vi "X-CAN_Connection_Stream_Connection.vi"() -> ()   [LabVIEW 2015]
uses:
  <vilib>/Stratom, Inc/X-CAN for myRIO (API)/X-CAN Class/Type Definitions/CAN_Speed.ctl
  <vilib>/Stratom, Inc/X-Modules for myRIO/Type Defs/MXPChannel.ctl
  <vilib>/Platform/TimedLoop/XDataNode/timing_clust.ctl
  <vilib>/Platform/TimedLoop/XDataNode/nitl_modes.ctl
  <vilib>/Platform/TimedLoop/XDataNode/wakeup.ctl
  <vilib>/platform/TimedLoop/XDataNode/XDataNode.xnode
  <vilib>/Stratom, Inc/X-CAN for myRIO (API)/X-CAN Class/X-CAN.lvclass
  <vilib>/Platform/TimedLoop/XDataNode/XDNodeRunTimeDep.lvlib
panel:
  out "Motor positions (degree)":T1(array[cluster]) {"Error Code (bits)" format="%b"}
  in  "Stop Button":bool
  # "REMEMBER: this subVI has always to be run as first."
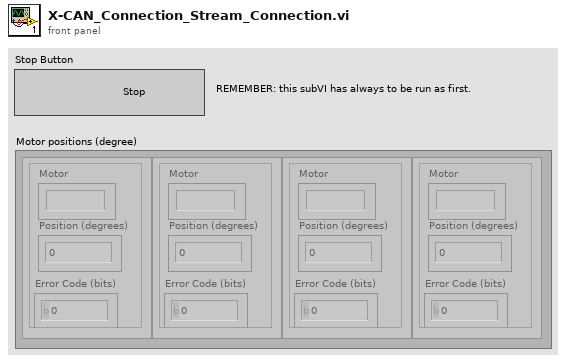
[diagram p1: front panel]
types:
  T1 = cluster{"Position (degrees)":i32, "Error Code (bits)":u8, "Motor":string}[]
  T2 = cluster{"Desired Position":u16, "Enable?":bool, "Reset?":bool}[]
  T3 = typedef "MXPChannel.ctl" = enum16{"A/MXP", "B/MXP"}
  T4 = typedef "X-CAN.lvclass/CAN_Speed.ctl" = u8
  T5 = cluster{"ID":u8, "Position":u16, "Error Code":u8}[]
  T6 = typedef "XDNodeRunTimeDep.lvlib/timing_clust.ctl" = cluster{"Expected End [f-1]":u64, "Actual End [f-1]":u64, "Finished Late? [f-1]":bool, "Expected End [i-1]":u64, "Actual End [i-1]":u64, "Finished Late? [i-1]":bool, "Expected Start [i]":u64, "Actual Start [i]":u64, "Expected Start [f]":u64, "Actual Start [f]":u64, "Source Name":string, "Structure Name":string, "Period":i64, "Deadline":i64, "Offset":i64, "Start":i64, "Priority":i32, "Timeout":i32, "Mode":T7, "Wakeup Reason":T8, "Error":errorcluster, "Source Type":string, "Secondary Source Type":string, "Global End Time":u64, "Global Start Time":u64, "Frame Duration":u64, "Iteration Duration":u64, "Assigned CPU":i32, "I/O Scan Engine Mode":u32}
  T7 = typedef "XDNodeRunTimeDep.lvlib/nitl_modes.ctl" = enum32{"No Change", "Process missed periods, maintain original phase", "Discard missed periods, maintain original phase", "Process missed periods, ignore original phase", "Discard missed periods, ignore original phase"}
  T8 = typedef "XDNodeRunTimeDep.lvlib/wakeup.ctl" = enum32{"Normal", "Aborted", "Asynchronous wakeup", "Timing source error", "Timed loop error", "Timeout"}
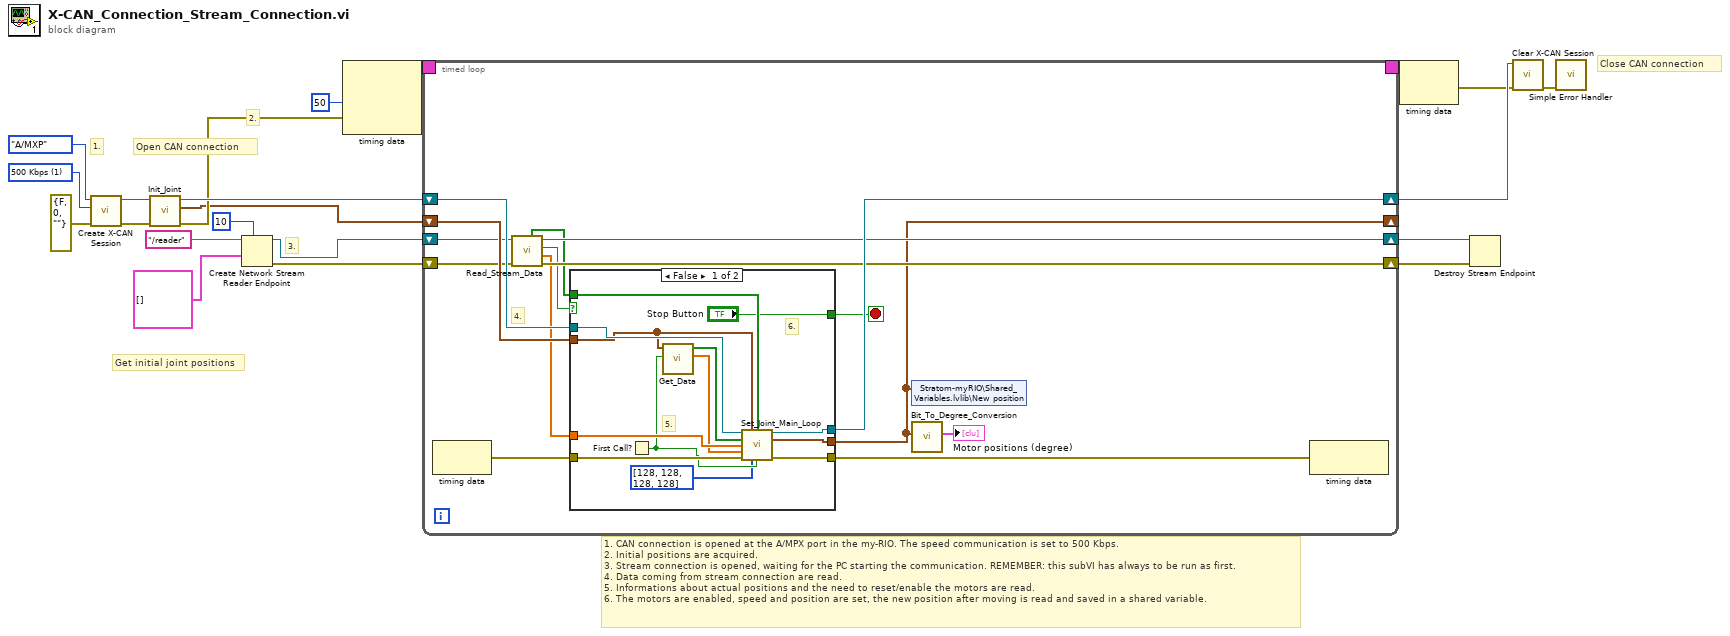
[diagram p0: block diagram]
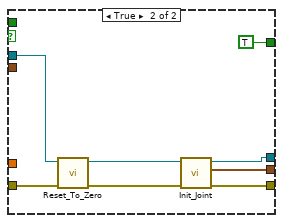
[diagram p2: hidden frame]
diagram:
  w20 = T4 1 items=["125 Kbps"=7, "250 Kbps"=3, "500 Kbps"=1, "1000 Kbps"=0, "95.238 Kbps"=6] ("CAN Speed [Kbps]")
  # "Close CAN connection"
  # "3."
  # "2."
  # "1."
  # "1. CAN connection is opened at the A/MPX port in the my-RIO. The speed communication is set to 500 Kbps.\n2. Initial positions are acquired.\n3. Stream connection is opened, waiting for the PC starting the communication. REMEMBER: this subVI has always to be run as first. \n4. Data coming from stream connection are read.\n5. Informations about actual positions and the need to reset/enable the motors are read.\n6. The motors are enabled, speed and position are set, the new position after moving is read and saved in a shared variable."
  # "Get initial joint positions"
  # "Open CAN connection"
  n1 = call <vilib>:"Create X-CAN Session.vi"("error in (no error)"=errorcluster {"status"=FALSE, "code"=0, "source"=""}, "CAN Speed [Kbps]"=w20, "MXP Channel"=MXPChannel."A/MXP") -> ("error out"=w11:errorcluster, "X-CAN Session out"=w12:refnum<class "X-CAN.lvclass">)  [unwired: 7 in]
  n2 = call "Init_Joint.vi"("error in"=w11, "X-CAN Session in"=w12) -> ("error out"=w9:errorcluster, "Init Position"=w8:T5, "X-CAN Session out"=w10:refnum<class "X-CAN.lvclass">)  [unwired: 5 in, 1 out]
  n3 = Create Network Stream Reader Endpoint(7:10 ("reader buffer size"), 9:T2 [] ("Commands 2"), 11:"/reader" ("reader name")) -> (0:w1:errorcluster, 3:w2:refnum<k21>)  [unwired: 4 in]
  n4 = node-c288(i64 50 ("Period"), w9) -> (w18:T6)  [unwired: 1 in]
  n5 = timed-loop {
    timing: w18 -> [_]
    timing-out: [_] -> w17
    shift-right: [w33] -> w15
    shift-left: w10 -> [w36]
    shift-right: [w23] -> _
    shift-left: w8 -> [w32]
    shift-right: [w27] -> w6
    shift-left: w1 -> [w29]
    shift-right: [w28] -> w5
    shift-left: w2 -> [w30]
    stop <- w31 stop-if-true
    # "4."
    n6 = node-c288() -> (w35:errorcluster)  [unwired: 1 in]
    n7 = call "Read_Stream_Data.vi"("error in (no error)"=w29, "Refnum in"=w30) -> ("error out"=w27:errorcluster, "Desired Position"=w24:dbl[], "Reset to zero position?"=w26:bool, "Refnum out"=w28:refnum<k21>, "Enabled motor?"=w25:bool[])  [unwired: 5 in]
    n8 = case shown="False" w26 {
      tunnel: w36 -> [w49 w57]
      tunnel: w35 -> [w48 w56]
      tunnel: [w47 w54] -> w34
      tunnel: [w46 w51] -> w33
      tunnel: [w45 w50] -> w23
      tunnel: w32 -> [w44 _]
      tunnel: ["Stop Button" TRUE ("stop")] -> w31
      tunnel: w25 -> [w42 _]
      tunnel: w24 -> [w41 _]
      frame False {
        # "6."
        # "5."
        n9 = First Call?() -> (First Call?: T/F=w38:bool)
        n10 = call "Get_Data.vi"("First Call?: T/F"=w38, "Init Position"=w44) -> ("Actual Positions"=w40:dbl[], "Reset Enable?"=w43:bool[])  [unwired: 8 in]
        n11 = call "Set_Joint_Main_Loop.vi"("X-CAN in"=w49, "Actual position"=w44, "Motor enabled?"=w42, "Reset?"=w43, "Desired position"=w41, "Current position"=w40, "error in (no error)"=w48, "Speed"=u16[] [128, 128, 128, 128], "Reset speed?"=w38) -> ("X-CAN out"=w46:refnum<class "X-CAN.lvclass">, "New position"=w45:T5, "error out"=w47:errorcluster)  [unwired: 4 in]
      }
      frame True {
        n12 = call "Reset_To_Zero.vi"("error in"=w56, "X-CAN Session in"=w57) -> ("error out"=w53:errorcluster, "X-CAN Session out"=w52:refnum<class "X-CAN.lvclass">)  [unwired: 8 in]
        n13 = call "Init_Joint.vi"("error in"=w53, "X-CAN Session in"=w52) -> ("error out"=w54:errorcluster, "Init Position"=w50:T5, "X-CAN Session out"=w51:refnum<class "X-CAN.lvclass">)  [unwired: 5 in, 1 out]
      }
    }
    n14 = shared-variable "Stratom-myRIO\\Shared_Variables.lvlib\\New position"(w23) -> ()  [unwired: 1 in, 1 out]
    n15 = call "Bit_To_Degree_Conversion.vi"("Actual joints positions"=w23) -> ("Motor positions (degree)"=→"Motor positions (degree)":T1)  [unwired: 10 in]
    n16 = node-c288(w34) -> ()  [unwired: 1 out]
  }
  n17 = node-c288(w17) -> (w13:errorcluster)
  n18 = Destroy Stream Endpoint(8:w6, 11:w5) -> ()  [unwired: 1 out]
  n19 = call <vilib>:"Clear X-CAN Session.vi"("error in (no error)"=w13, "X-CAN Session in"=w15) -> ("error out"=w14:errorcluster)  [unwired: 9 in]
  n20 = call <vilib>:"Simple Error Handler.vi"("error in (no error)"=w14) -> ()  [unwired: 4 in, 5 out]
